vi "IRISS V2 Stage Ref Follow.vi"(6 "Stage Cmd Posit":dbl[](array[numeric]), 7 "Left or Right Arm":i32(ring)=1 items=["Left Arm", "Right Arm"]) -> (2 "Stage Out Posit":dbl[](array[numeric]))   [LabVIEW 2016]
uses:
  EyeRobotDLL.dll
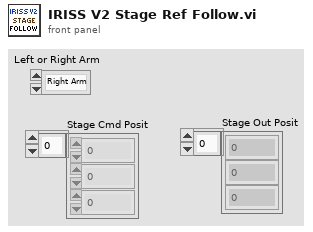
[diagram p1: front panel]
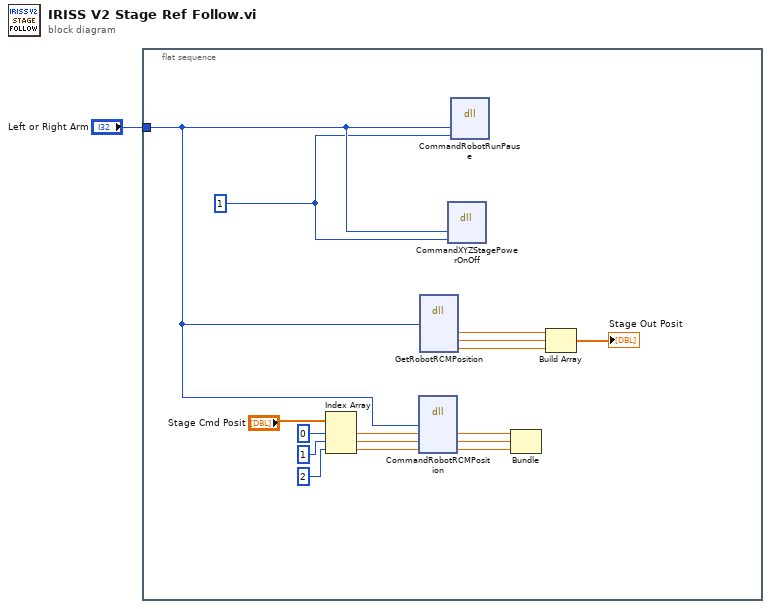
[diagram p0: block diagram]
diagram:
  n1 = flat-sequence {
    tunnel: "Left or Right Arm" -> [w3]
    frame #0 {
      w2 = 1 ("OnOff")
      n2 = Index Array(array="Stage Cmd Posit", index #1=0 ("index"), index #2=1 ("index"), index #3=2 ("index")) -> (element #1=w11:dbl, element #2=w10:dbl, element #3=w9:dbl)
      n3 = dll-call lib="D:/IRISSoft LV2016 beta/Host Demo/Functions/EyeRobotDLL.dll" fn="CommandRobotRCMPosition"("id"=w3, "x"=w11, "y"=w10, "z"=w9) -> ("x"=w15:dbl, "y"=w16:dbl, "z"=w17:dbl)  [unwired: 5 in, 2 out]
      n4 = dll-call lib="D:/IRISSoft LV2016 beta/Host Demo/Functions/EyeRobotDLL.dll" fn="GetRobotRCMPosition"("id"=w3) -> ("x"=w7:dbl, "y"=w6:dbl, "z"=w5:dbl)  [unwired: 8 in, 2 out]
      n5 = dll-call lib="D:/IRISSoft LV2016 beta/Host Demo/Functions/EyeRobotDLL.dll" fn="CommandXYZStagePowerOnOff"("id"=w3, "OnOff"=w2) -> ()  [unwired: 6 in, 2 out]
      n6 = dll-call lib="D:/IRISSoft LV2016 beta/Host Demo/Functions/EyeRobotDLL.dll" fn="CommandRobotRunPause"("id"=w3, "RunPause"=w2) -> ()  [unwired: 6 in, 2 out]
      n7 = Bundle("x"=w15, "y"=w16, "z"=w17) -> ()  [unwired: 1 in, 1 out]
      n8 = Build Array(w7, w6, w5) -> (→"Stage Out Posit":dbl[])
    }
  }
